vi "Config Setpoint.vi"(0 "VISA resource name":refnum<visa-resource-name>, 5 "Loop (0: 1)":u16(ring) items=["1", "2"], 7 "Setpoint (0.0)":dbl min=-273.0 max=300000.0 step=0.0001 format="%.4f", 11 "error in (no error)":errorcluster) -> (4 "VISA resource name out":refnum<visa-resource-name>, 15 "error out":errorcluster)   [LabVIEW 2019, in "Lake Shore Cryotronics 340.lvlib"]
doc: "This VI Configures a control loop's setpoint."
uses:
  Lake Shore Cryotronics 340.lvlib
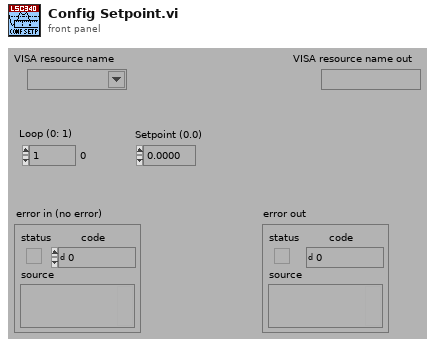
[diagram p1: front panel]
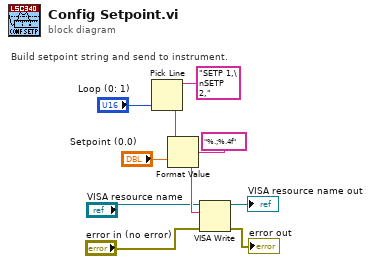
[diagram p0: block diagram]
diagram:
  # "Build setpoint string and send to instrument."
  n1 = Pick Line(multi-line string="SETP 1,\nSETP 2,", line index="Loop (0: 1)") -> (output string=w8:string)  [unwired: 1 in]
  n2 = Format Value(string ("")=w8, format string="%.;%.4f", value (0)="Setpoint (0.0)") -> (output string=w5:string)
  n3 = VISA Write(VISA resource name="VISA resource name", write buffer=w5, error in (no error)="error in (no error)") -> (VISA resource name out=→"VISA resource name out":refnum<visa-resource-name>, error out=→"error out":errorcluster)  [unwired: 1 out]
